vi "Needle Valve labVIEW Code.vi"() -> ()   [LabVIEW 2025]
uses:
  modesEnum.ctl
  <vilib>/Utility/file.llb/Read Delimited Spreadsheet (DBL).vi
  <vilib>/gmath/NI_Gmath.lvlib
  d3b0afdc-d7ac-4f1a-8ecc-0aeb21fe1e80.vi
  c8945bc9-af31-4a2e-9b52-27840c61c0f1.vi
  PIDController/PIDController.lvclass
  e7797c04-791b-4eea-89a1-5a3bec2431d3.vi
  bf5fd3a0-ddf8-478e-bb95-a39885d33854.vi
  0890acf7-df83-934e-a7ac-ae51bc85d557.vi
  d872897a-af24-4a4d-87bc-a1bb59a840a8.vi
  0285ecf2-4d18-4427-ace1-61b1951a0741.vi
  <vilib>/Instr/_visa.llb/VISA Configure Serial Port (Instr).vi
  <vilib>/Utility/file.llb/Write Delimited Spreadsheet (string).vi
  spikeController/spikeController.lvclass
panel:
  out "last error":dbl
  in  "Use D1":bool
  in  "Use D2":bool
  in  "Use Avg":bool
  in  "Save Graphs":bool
  in  "Set setPoint":dbl format="%.3f"
  in  "Set Spike Position":dbl format="%.3f"
  in  "setPoint":dbl(knob) scale=0.0..1000.0
  in  "A_max":dbl=6.5
  in  "A_min":dbl
  in  "k_i":dbl
  in  "k_d":dbl
  in  "k_p":dbl
  out "SafetyClose":bool
  out "PID":bool
  out "Manual":bool
  out "Idle":bool
  out "Ducer1":bool
  out "Ducer2":bool
  out "Avg Ducers":bool
  out "Read Pressure Ducer":dbl
  out "Raw Pressure Ducer 2":dbl
  in  "spikeController.lvclass":refnum<class "spikeController.lvclass">
  out "underAmin":bool
  out "overAmax":bool
  out "PID Output":dbl[](graph)
  out "PID Translated Output":dbl
  out "PID Output":dbl
  in  "loop stop 2":bool
  in  "loop stop 1":bool
  in  "PIDController.lvclass":refnum<class "PIDController.lvclass">
  out "VISA resource name out":refnum<visa-resource-name>
  in  "?":u32(colorbox)
  out "Reading Pressure Sensor":dbl[](graph)
  in  "?":dbl
  out "Motor Signal":string
  in  "stop program":bool
  in  "return spike":bool
  out "Spike Position \n(via Potentiometer)":dbl[](graph)
  out "Arduino Error":errorcluster
  in  "VISA resource Port":refnum<visa-resource-name>
  out "distance to go":dbl caption="Distance to Go (in)\n(For Reference Only)" format="%.3f"
  out "spike position":dbl format="%.3f"
  in  "Set Spike Position (in)":dbl(slide) scale=0.0..6.8
  out "?":dbl(slide) scale=0.0..1000.0
  out "Stagnation Flow Temp (K)\n(For Refrence only)":dbl
  out "Raw Pressure Ducer":dbl
  in  "Sensor Offsets":dbl[](array[numeric])=[10.0, 10.0, 0.0, 22.0]
  in  "Sensor K-values":dbl[](array[numeric])=[10.0, 10.0, 0.0, 22.0]
  in  "Exit PID Mode":bool
  in  "manual exit button":bool
  in  "Motor Control Loop Rate (ms)":dbl
  out "Set Motor RPM":dbl(knob) scale=0.0..200.0
  in  "PID Mode":bool
  in  "Manual Positioning Mode":bool
  in  "Stop Sensors":bool
  in  "Sensor Loop Rate (ms)":dbl
  out "Time Since Start (s)\n(For Reference Only)":dbl format="%.2f"
  in  "Start Sensors":bool
  in  "Load Inputs":bool
  in  "Save Inputs":bool
  out "Potentiometer distance":dbl
  out "Port":i32
  out "ConnectionType":i32
  out "DeviceType":i32
  out "Labjack error":errorcluster
  # "34HS59-6004S Motor Torque Curve (For Reference)"
  # "Labjack/Arduino Resources"
  # "Inputs and LabJack Sensor Monitors"
  # "PID Inputs"
  # "Motor RPM >200 RPM"
  # "Potentiometer"
  # "Inefficent Torque for High Mass Flow/Thrust Tests"
  # "Ducer"
  # "Thermocouple"
  # "Motor RPM < 200 RPM"
  # "(Labjack Auto-Populates)"
  # "(dial indicator for range reference)"
  # "COM Port for Arduino"
  # "Stop sensors automatically saves sensor data"
  # "Needliest"
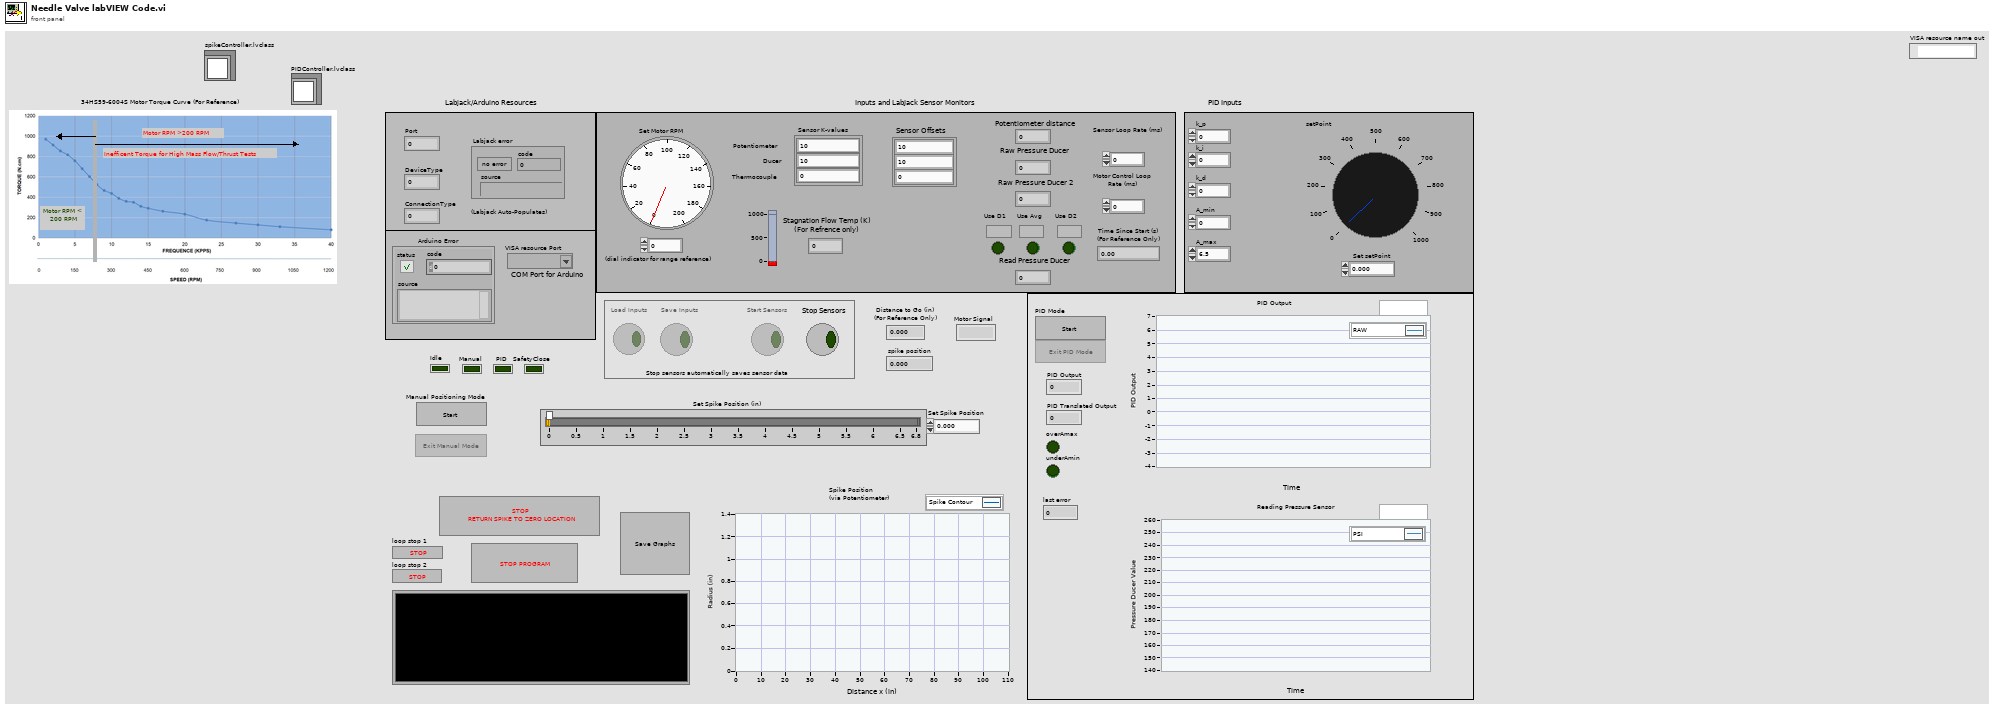
[diagram p1: front panel]
types:
  T1 = typedef "modesEnum.ctl" = enum16{"SafetyOpen", "SafetyClose", "SaveFile", "PIDControl", "ManualControl", "Idle"}
  T2 = enum8{"Enabled", "Disabled", "Disabled and Grayed Out"}
  T3 = enum16{"Potentiometer", "Ducer", "Thermocouple", "Ducer2"}
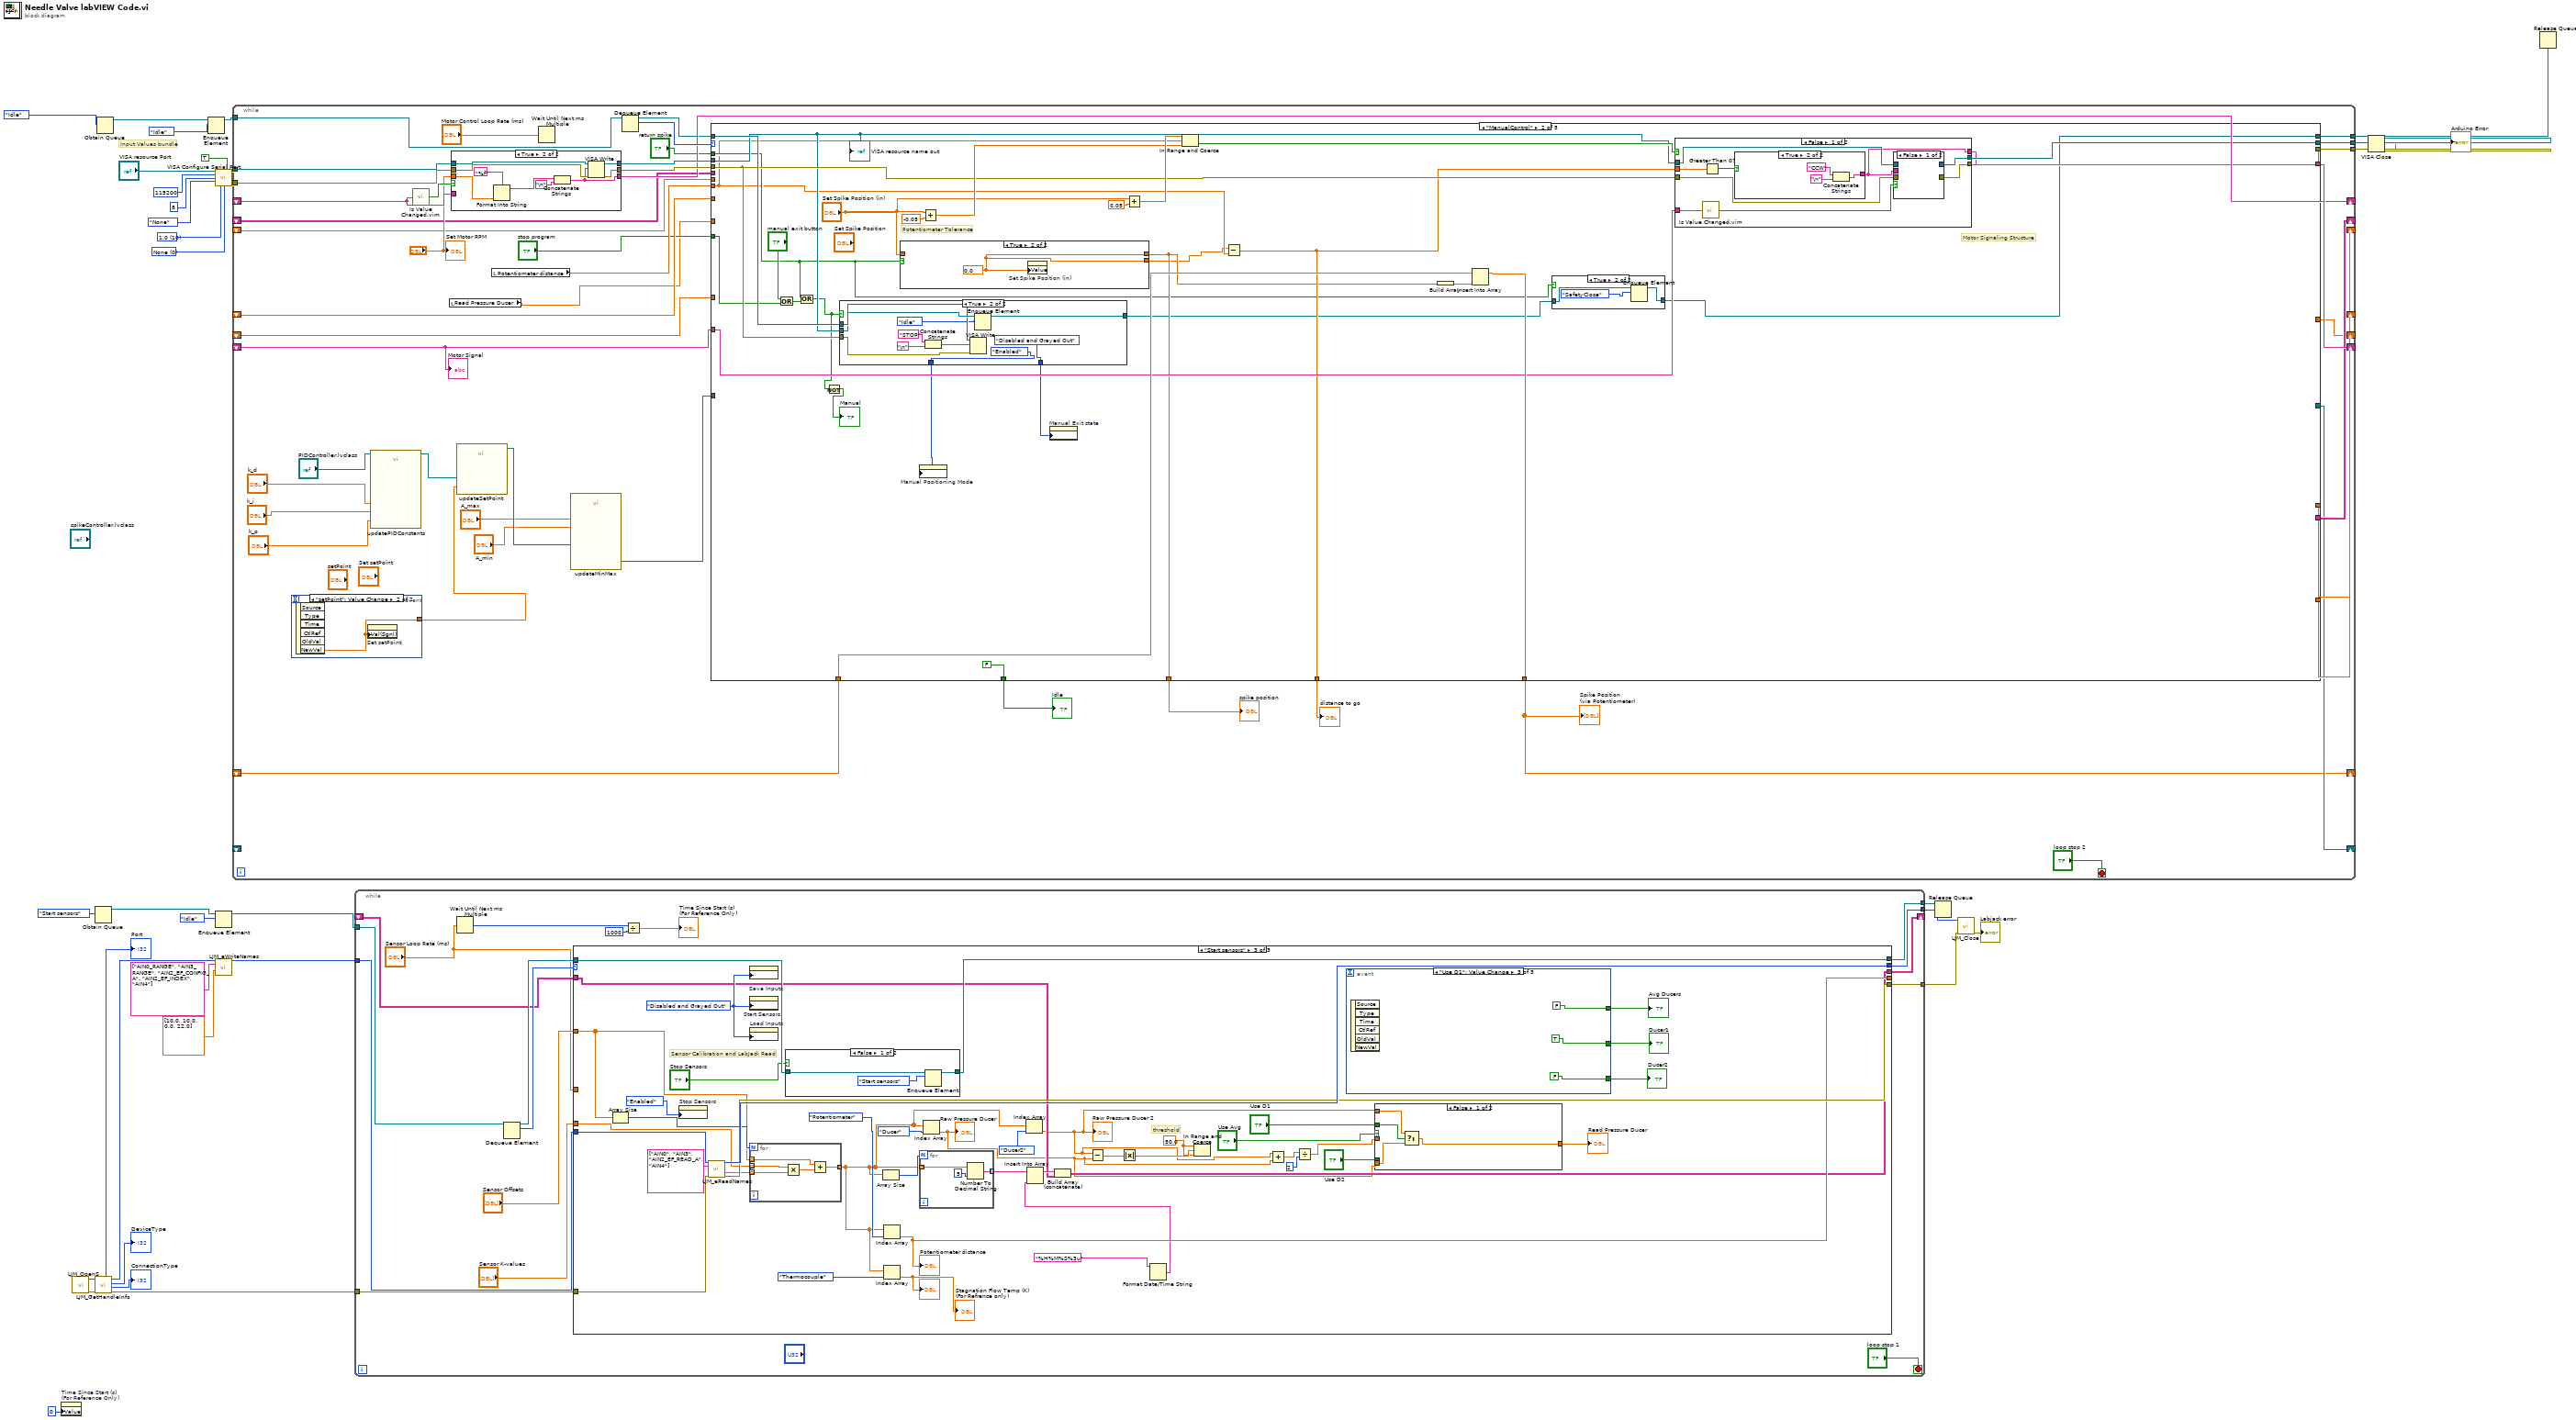
[diagram p0: block diagram]
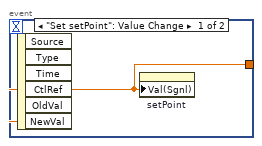
[diagram p2: hidden frame]
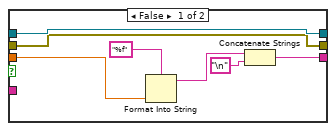
[diagram p3: hidden frame]
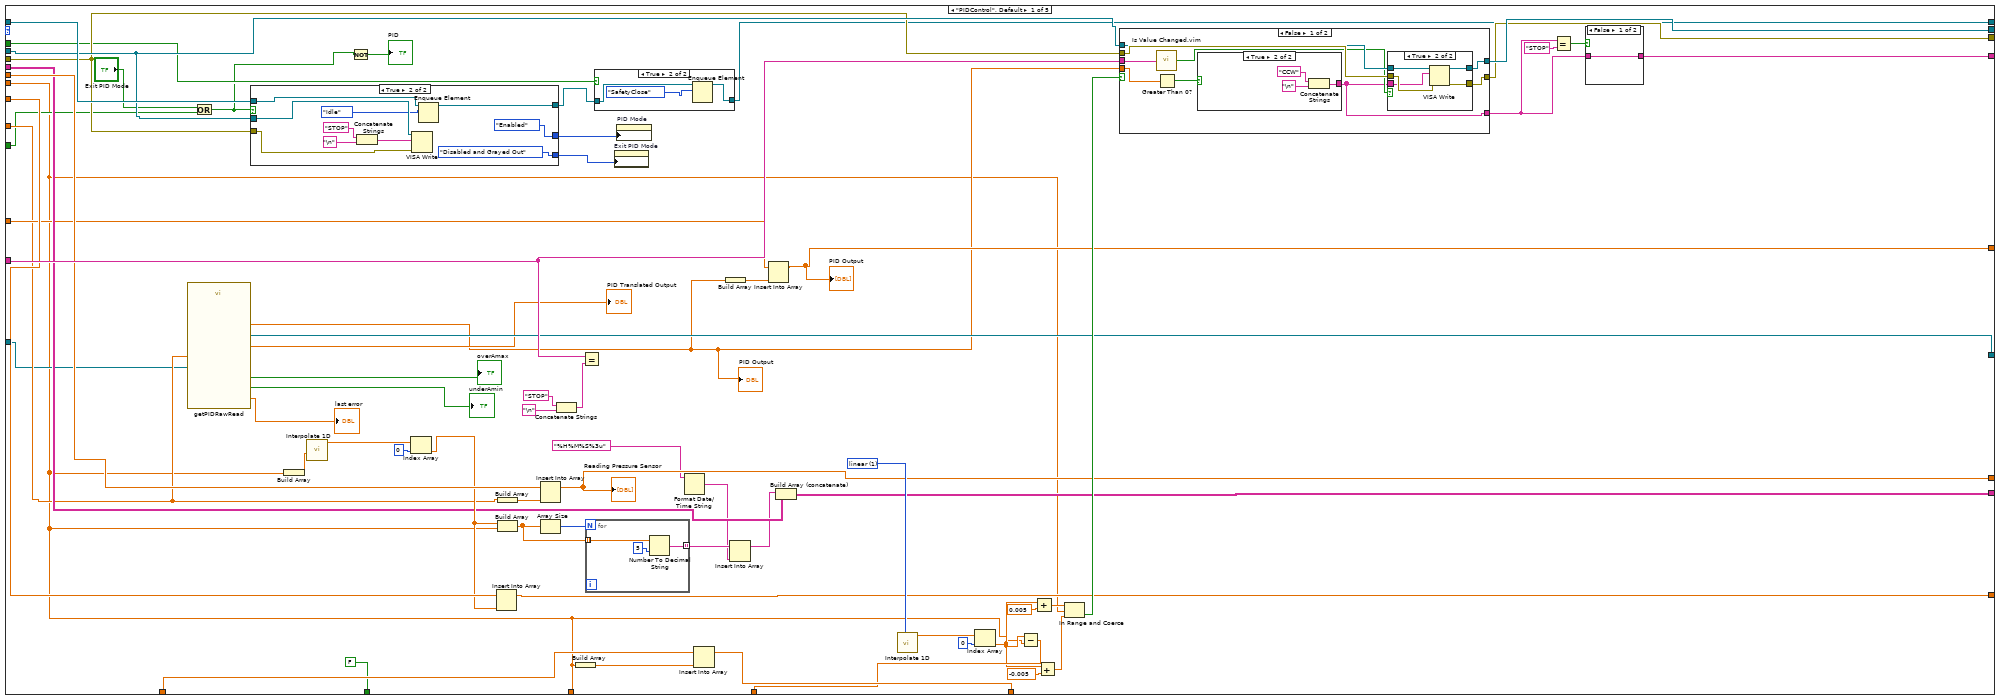
[diagram p4: hidden frame]
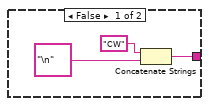
[diagram p8: hidden frame]
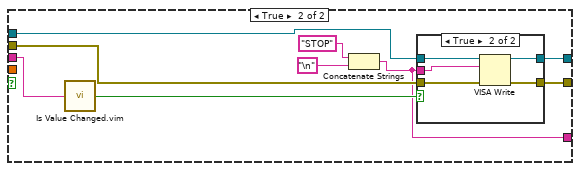
[diagram p9: hidden frame]
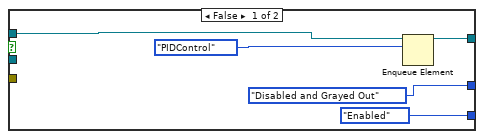
[diagram p11: hidden frame]
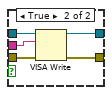
[diagram p14: hidden frame]
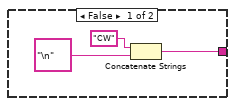
[diagram p15: hidden frame]
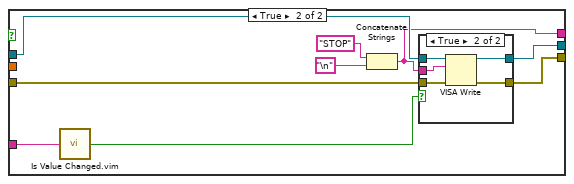
[diagram p16: hidden frame]
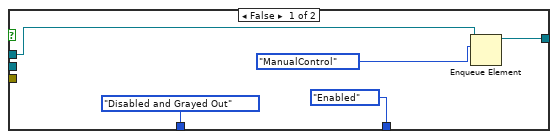
[diagram p18: hidden frame]
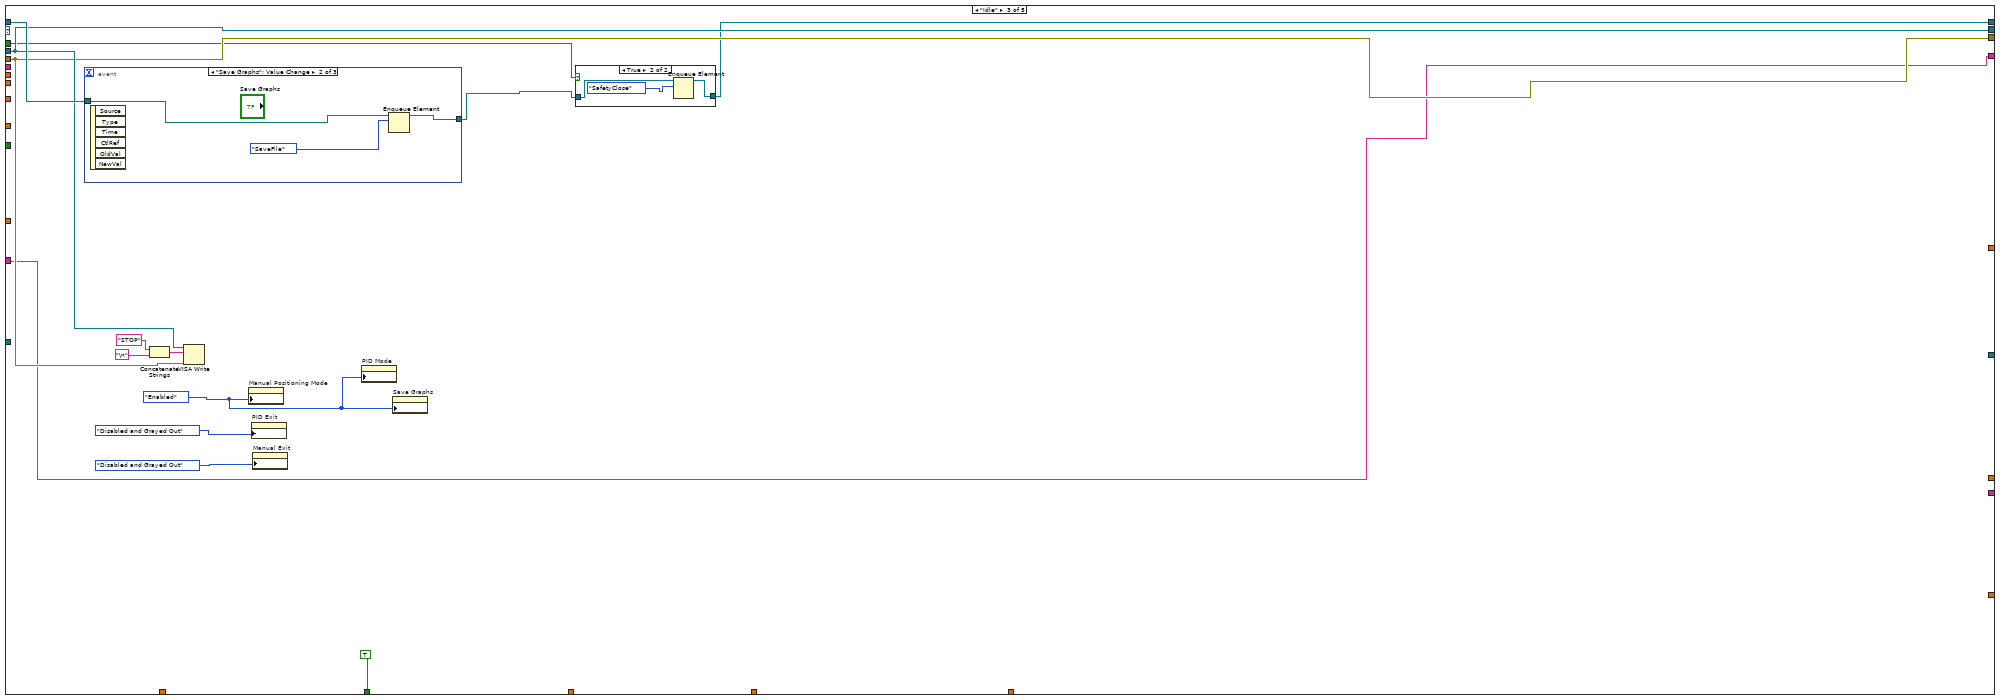
[diagram p19: hidden frame]
diagram:
  w6 = u16 0 items=["None", "XON/XOFF", "RTS/CTS", "XON/XOFF & RTS/CTS", "DTR/DSR", "XON/XOFF & DTR/DSR"] ("flow control (0:none)")
  w7 = u16 10 items=["1.0"=10, "1.5"=15, "2.0"=20] ("stop bits (10: 1 bit)")
  # "Input Values bundle"
  n1 = property on="Time Since Start (s)\n(For Reference Only)" class="DigNum (strict)"("Value"=u32 0 ("Time Since Start (s)\n(For Reference Only) 2")) -> ()  [unwired: 2 in, 2 out]
  n2 = call "LJM_OpenS.vi"() -> ("error out"=w31:errorcluster, "Handle"=w35:i32)  [unwired: 10 in]
  n3 = Obtain Queue(element data type=enum16{"Start sensors", "load Values", "Idle"}."Start sensors" ("Enum")) -> (queue out=w25:refnum<queue>)  [unwired: 4 in, 2 out]
  n4 = call "LJM_GetHandleInfo.vi"("error in"=w31, "Handle In"=w35) -> ("error out"=w30:errorcluster, "ConnectionType"=→"ConnectionType":i32, "DeviceType"=→"DeviceType":i32, "Handle Out"=w18:i32, "Port"=→"Port":i32)  [unwired: 2 in, 3 out]
  n5 = Obtain Queue(element data type=modesEnum."Idle" ("modesEnum")) -> (queue out=w27:refnum<queue>)  [unwired: 4 in, 2 out]
  n6 = Enqueue Element(queue=w27, element=modesEnum."Idle" ("modesEnum")) -> (queue out=w26:refnum<queue>)  [unwired: 2 in, 2 out]
  n7 = call-poly "VISA Configure Serial Port"("VISA resource name"="VISA resource Port", "Enable Termination\nChar (T)"=TRUE ("Enable Termination\nChar (T)"), "baud rate (9600)"=u32 115200, "data bits (8)"=u16 8, "parity (0:none)"=enum16{"None", "Odd", "Even", "Mark", "Space"}."None", "stop bits (10: 1 bit)"=w7, "flow control (0:none)"=w6) -> ("VISA resource name out"=w4:refnum<visa-resource-name>, "error out"=w5:errorcluster)  [unwired: 7 in]
  n8 = Enqueue Element(queue=w25, element=enum16{"Start sensors", "load Values", "Idle"}."Idle" ("Enum")) -> (queue out=w24:refnum<queue>)  [unwired: 2 in, 2 out]
  n9 = call "LJM_eWriteNames.vi"("Handle In"=w18, "aNames"=string[] ["AIN0_RANGE", "AIN3_RANGE", "AIN2_EF_CONFIG_A", "AIN2_EF_INDEX", "AIN4"], "aValuesIn"=dbl[] [10.0, 10.0, 0.0, 22.0]) -> ("Handle Out"=w17:i32)  [unwired: 10 in, 2 out]
  n10 = while {
    tunnel: w26 -> [w82]
    tunnel: [w80] -> w21
    tunnel: [w77] -> w12
    tunnel: [w76] -> w11
    shift-right: [w75] -> _
    shift-left: _ -> [w74]
    tunnel: w5 -> [w73]
    tunnel: w4 -> [w72]
    shift-right: [w68] -> _
    shift-left: _ -> [w67]
    shift-right: [w59] -> _
    shift-left: _ -> [_]
    shift-right: [w64] -> _
    shift-left: _ -> [w63]
    shift-right: [w62] -> _
    shift-left: _ -> [w57]
    shift-right: [w61] -> _
    shift-left: _ -> [w60]
    shift-right: [w55] -> _
    shift-left: _ -> [w56]
    shift-right: [w52] -> _
    shift-left: _ -> [w53]
    stop <- "loop stop 2" stop-if-true
    n11 = event shown="[1] \"setPoint\": Value Change" {
      selector: _ -> [_ _]
      dyn-events: _ -> [_ _]
      timeout: _ -> [_ _]
      tunnel: [w83 w84] -> w37
      event "Set setPoint": Value Change {
        n12 = event-data() -> ("NewVal"=w83:dbl)  [unwired: 1 in, 5 out]
        n13 = property on="setPoint" class="Knob (strict)"("Val(Sgnl)"=w83) -> ()  [unwired: 2 in, 2 out]
      }
      event "setPoint": Value Change {
        n14 = event-data() -> ("NewVal"=w84:dbl)  [unwired: 1 in, 5 out]
        n15 = property on="Set setPoint" class="DigNum (strict)"("Val(Sgnl)"=w84) -> ()  [unwired: 2 in, 2 out]
      }
    }
    n16 = call "updatePIDConstants.vi"("new k_d"="k_d", "new k_p"="k_p", "new k_i"="k_i", "PIDController in"="PIDController.lvclass") -> ("PIDController out"=w47:refnum<class "PIDController.lvclass">)  [unwired: 6 in, 1 out]
    n17 = call "Is Value Changed.vim"("value"=w67) -> ("changed or first call?"=w69:bool)
    n18 = local read "Read Pressure Ducer"() -> (w38:dbl)
    n19 = case shown="True" w69 {
      tunnel: w73 -> [w90 w100]
      tunnel: [w86 w92] -> w68
      tunnel: w72 -> [w91 w99]
      tunnel: [w90 w98] -> w71
      tunnel: [w91 w95] -> w70
      tunnel: "?" -> [w89 w97]
      tunnel: w67 -> [_ _]
      frame False {
        n20 = Format Into String(format string="%f", w89) -> (resulting string=w87:string)  [unwired: 2 in, 1 out]
        n21 = Concatenate Strings(w87, "\n" ("string")) -> (w86:string)
      }
      frame True {
        n22 = Format Into String(format string="%f", w97) -> (resulting string=w94:string)  [unwired: 2 in, 1 out]
        n23 = Concatenate Strings(w94, "\n" ("string")) -> (w92:string)
        n24 = VISA Write(VISA resource name=w99, write buffer=w92, error in (no error)=w100) -> (VISA resource name out=w95:refnum<visa-resource-name>, error out=w98:errorcluster)  [unwired: 1 out]
      }
    }
    n25 = call "updateSetPoint.vi"("new setpoint"=w37, "PIDController in"=w47) -> ("PIDController out"=w48:refnum<class "PIDController.lvclass">)  [unwired: 8 in, 1 out]
    n26 = local read "Potentiometer distance"() -> (w78:dbl)
    n27 = Wait Until Next ms Multiple(millisecond multiple="Motor Control Loop Rate (ms)") -> ()  [unwired: 1 out]
    n28 = call "updateMinMax.vi"("a_max"="A_max", "a_min"="A_min", "PIDController in"=w48) -> ("PIDController out"=w45:refnum<class "PIDController.lvclass">)  [unwired: 7 in, 1 out]
    n29 = Dequeue Element(queue=w82) -> (queue out=w49:refnum<queue>, element=w81:T1)  [unwired: 2 in, 2 out]
    n30 = case shown="\"ManualControl\"" w81 {
      tunnel: [w111 w231 w314 w347 _] -> w80
      tunnel: w49 -> [w165 w254 w323 w346 _]
      tunnel: w78 -> [w107 w230 _ w341 _]
      tunnel: w70 -> [w154 w243 w317 w351 _]
      tunnel: [w157 w248 w317 w349 _] -> w77
      tunnel: w71 -> [w153 w245 w316 w352 _]
      tunnel: [w156 w247 w316 w348 _] -> w76
      tunnel: [w150 w246 w315 w350 _] -> w75
      tunnel: w74 -> [w148 w236 w315 w340 _]
      tunnel: "return spike" -> [w110 w233 w312 w339 _]
      tunnel: [w140 _ _ _ _] -> w64
      tunnel: w63 -> [w141 _ _ _ _]
      tunnel: [w138 _ _ _ _] -> w62
      tunnel: w57 -> [w137 _ _ _ w399]
      tunnel: [w134 _ _ _ _] -> w61
      tunnel: w60 -> [w133 _ _ _ _]
      tunnel: w38 -> [w121 _ _ _ _]
      tunnel: w45 -> [w109 _ _ _ _]
      tunnel: [w127 _ _ _ _] -> w59
      tunnel: w56 -> [w125 _ _ _ w398]
      tunnel: [w124 _ _ _ _] -> w55
      tunnel: "stop program" -> [w117 w241 _ _ _]
      tunnel: w53 -> [w115 w238 _ w345 w419]
      tunnel: [w114 w237 _ w344 _] -> w52
      tunnel: [w113 w235 _ w343 _] -> w51
      tunnel: [w107 w234 _ w342 _] -> w50
      tunnel: [FALSE FALSE TRUE FALSE FALSE] -> w39
      frame "PIDControl", Default {
        w158 = 1 items=["nearest", "linear", "spline", "cubic Hermite", "Lagrange"] ("method")
        n31 = call "getPIDRawRead.vi"("sensorValue"=w121, "PIDController in"=w109) -> ("overAmin"=→"underAmin":bool, "translatedPIDOutput"=→"PID Translated Output":dbl, "PIDRawRead"=w123:dbl, "PIDController out"=w127:refnum<class "PIDController.lvclass">, "underAmax"=→"overAmax":bool, "lastErrorRead"=→"last error":dbl)  [unwired: 4 in]
        "PID Output" <- w123
        n32 = Or(x="Exit PID Mode", y=w117) -> (x .or. y?=w106:bool)
        n33 = case shown="True" w106 {
          tunnel: w165 -> [w213 w223]
          tunnel: [w212 w222] -> w112
          tunnel: w154 -> [_ w218]
          tunnel: w153 -> [_ w217]
          tunnel: [T2."Disabled and Grayed Out" ("Disabled") T2."Enabled" ("Disabled")] -> w103
          tunnel: [T2."Enabled" ("Disabled") T2."Disabled and Grayed Out" ("Disabled")] -> w102
          frame False {
            n34 = Enqueue Element(queue=w213, element=modesEnum."PIDControl" ("modesEnum")) -> (queue out=w212:refnum<queue>)  [unwired: 2 in, 2 out]
          }
          frame True {
            n35 = Concatenate Strings("STOP" ("write buffer"), "\n" ("write buffer")) -> (w221:string)
            n36 = VISA Write(VISA resource name=w218, write buffer=w221, error in (no error)=w217) -> ()  [unwired: 3 out]
            n37 = Enqueue Element(queue=w223, element=modesEnum."Idle" ("modesEnum")) -> (queue out=w222:refnum<queue>)  [unwired: 2 in, 2 out]
          }
        }
        n38 = Build Array(w107) -> (w147:dbl[])
        n39 = call <vilib>:"Interpolate 1D.vi"("xi"=w147) -> ("yi"=w146:dbl[])  [unwired: 8 in, 2 out]
        n40 = Not(x=w106) -> (.not. x?=→"PID":bool)
        n41 = Index Array(array=w146, index=0) -> (element=w136:dbl)
        n42 = Insert Into Array(array=w141, new element=w136) -> (w140:dbl[])  [unwired: 1 in]
        n43 = Build Array(w121) -> (w139:dbl[])
        n44 = Build Array(w136, w107) -> (w132:dbl[])
        n45 = Insert Into Array(array=w137, new element=w139) -> (w138:dbl[])  [unwired: 1 in]
        "Reading Pressure Sensor" <- w138
        n46 = Array Size(array=w132) -> (size(s)=w131:i32)
        n47 = Concatenate Strings("STOP" ("string"), "\n" ("string")) -> (w142:string)
        n48 = Build Array(w107) -> (w116:dbl[])
        n49 = Equal?(x=w148, y=w142) -> ()  [unwired: 1 out]
        n50 = for {
          N: w131 -> [_]
          tunnel: w132 -> [w172] mode=indexing
          tunnel: [w170] -> w135 mode=indexing
          n51 = Number To Decimal String(number=w172, width (-)=i16 5) -> (decimal integer string=w170:string)
        }
        n52 = case shown="True" w110 {
          tunnel: w112 -> [w166 w169]
          tunnel: [w166 w168] -> w111
          frame False {
          }
          frame True {
            n53 = Enqueue Element(queue=w169, element=modesEnum."SafetyClose" ("modesEnum")) -> (queue out=w168:refnum<queue>)  [unwired: 2 in, 2 out]
          }
        }
        n54 = property on="Exit PID Mode" class="Bool"("DisabledEnum"=w102) -> ()  [unwired: 2 in, 2 out]
        n55 = property on="PID Mode" class="Bool"("DisabledEnum"=w103) -> ()  [unwired: 2 in, 2 out]
        n56 = Format Date/Time String(time format string (%c)="%H%M%S%3u") -> (date/time string=w128:string)  [unwired: 2 in]
        n57 = Insert Into Array(array=w115, new element=w116) -> (w114:dbl[])  [unwired: 1 in]
        n58 = Build Array(w123) -> (w122:dbl[])
        n59 = Insert Into Array(array=w135, new element=w128) -> (w130:string[])  [unwired: 1 in]
        n60 = Insert Into Array(array=w125, new element=w122) -> (w124:dbl[])  [unwired: 1 in]
        "PID Output" <- w124
        n61 = Build Array (concatenate)(w130, w133) -> (w134:string[][])
        n62 = call <vilib>:"Interpolate 1D.vi"("method"=w158) -> ("yi"=w159:dbl[])  [unwired: 8 in, 2 out]
        n63 = Index Array(array=w159, index=0) -> (element=w108:dbl)
        n64 = Subtract(x=w108, y=w107) -> (x-y=w113:dbl)
        n65 = Add(x=w108, y=0.005) -> (x+y=w164:dbl)
        n66 = Add(x=w108, y=-0.005) -> (x+y=w162:dbl)
        n67 = In Range and Coerce(upper limit=w164, x=w107, lower limit=w162) -> (In Range?=w155:bool)  [unwired: 1 out]
        n68 = case shown="False" w155 {
          tunnel: w123 -> [w182 _]
          tunnel: w154 -> [w180 w203]
          tunnel: [w178 w200] -> w157
          tunnel: w153 -> [w181 w199]
          tunnel: [w179 w198] -> w156
          tunnel: [w175 w195] -> w151
          tunnel: w148 -> [w177 w202]
          frame False {
            n69 = call "Is Value Changed.vim"("value"=w177) -> ("changed or first call?"=w176:bool)
            n70 = Greater Than 0?(x=w182) -> (x > 0?=w183:bool)
            n71 = case shown="True" w183 {
              tunnel: [w189 w192] -> w175
              frame False {
                n72 = Concatenate Strings("CW" ("write buffer"), "\n" ("write buffer")) -> (w189:string)
              }
              frame True {
                n73 = Concatenate Strings("CCW" ("write buffer"), "\n" ("write buffer")) -> (w192:string)
              }
            }
            n74 = case shown="True" w176 {
              tunnel: w181 -> [_ w188]
              tunnel: w180 -> [_ w187]
              tunnel: [_ w186] -> w179
              tunnel: [_ w185] -> w178
              tunnel: w175 -> [_ w184]
              frame False {
              }
              frame True {
                n75 = VISA Write(VISA resource name=w187, write buffer=w184, error in (no error)=w188) -> (VISA resource name out=w185:refnum<visa-resource-name>, error out=w186:errorcluster)  [unwired: 1 out]
              }
            }
          }
          frame True {
            n76 = call "Is Value Changed.vim"("value"=w202) -> ("changed or first call?"=w201:bool)
            n77 = Concatenate Strings("STOP" ("write buffer"), "\n" ("write buffer")) -> (w195:string)
            n78 = case shown="True" w201 {
              tunnel: w195 -> [_ w208]
              tunnel: w203 -> [_ w207]
              tunnel: [_ w206] -> w200
              tunnel: w199 -> [_ w205]
              tunnel: [_ w204] -> w198
              frame False {
              }
              frame True {
                n79 = VISA Write(VISA resource name=w207, write buffer=w208, error in (no error)=w205) -> (VISA resource name out=w206:refnum<visa-resource-name>, error out=w204:errorcluster)  [unwired: 1 out]
              }
            }
          }
        }
        n80 = Equal?(x=w151, y="STOP" ("write buffer")) -> (x = y?=w149:bool)
        n81 = case shown="False" w149 {
          tunnel: [w173 w174] -> w150
          tunnel: w151 -> [w173 w174]
          frame False {
          }
          frame True {
          }
        }
      }
      frame "ManualControl" {
        # "Motor Signaling Structure"
        # "Potentiometer Tolerance"
        n82 = Or(x="manual exit button", y=w241) -> (x .or. y?=w240:bool)
        n83 = Or(x=w233, y=w240) -> (x .or. y?=w228:bool)
        n84 = Not(x=w228) -> (.not. x?=→"Manual":bool)
        n85 = case shown="True" w228 {
          tunnel: w254 -> [w299 w309]
          tunnel: [w298 w308] -> w232
          tunnel: w243 -> [_ w304]
          tunnel: w245 -> [_ w303]
          tunnel: [T2."Enabled" ("Disabled") T2."Disabled and Grayed Out" ("Disabled")] -> w225
          tunnel: [T2."Disabled and Grayed Out" ("Disabled") T2."Enabled" ("Disabled")] -> w224
          frame False {
            n86 = Enqueue Element(queue=w299, element=modesEnum."ManualControl" ("modesEnum")) -> (queue out=w298:refnum<queue>)  [unwired: 2 in, 2 out]
          }
          frame True {
            n87 = Concatenate Strings("STOP" ("write buffer"), "\n" ("write buffer")) -> (w307:string)
            n88 = VISA Write(VISA resource name=w304, write buffer=w307, error in (no error)=w303) -> ()  [unwired: 3 out]
            n89 = Enqueue Element(queue=w309, element=modesEnum."Idle" ("modesEnum")) -> (queue out=w308:refnum<queue>)  [unwired: 2 in, 2 out]
          }
        }
        n90 = case shown="True" w233 {
          tunnel: [w259 w260] -> w229
          tunnel: "Set Spike Position (in)" -> [w259 _]
          tunnel: [w259 w260] -> w234
          frame False {
          }
          frame True {
            w260 = 0.0
            n91 = property on="Set Spike Position (in)" class="Slide (strict)"("Value"=w260) -> ()  [unwired: 2 in, 2 out]
          }
        }
        n92 = property on="Manual Positioning Mode" class="Bool"("DisabledEnum"=w224) -> ()  [unwired: 2 in, 2 out]
        n93 = Add(x="Set Spike Position (in)", y=-0.05) -> (x+y=w250:dbl)
        n94 = property on="Manual Exit state" class="Bool"("DisabledEnum"=w225) -> ()  [unwired: 2 in, 2 out]
        n95 = Add(x="Set Spike Position (in)", y=0.05) -> (x+y=w252:dbl)
        n96 = In Range and Coerce(upper limit=w252, x=w230, lower limit=w250) -> (In Range?=w253:bool)  [unwired: 1 out]
        n97 = Subtract(x=w229, y=w230) -> (x-y=w235:dbl)
        n98 = Build Array(w234) -> (w239:dbl[])
        n99 = Insert Into Array(array=w238, new element=w239) -> (w237:dbl[])  [unwired: 1 in]
        n100 = case shown="True" w233 {
          tunnel: w232 -> [w255 w258]
          tunnel: [w255 w257] -> w231
          frame False {
          }
          frame True {
            n101 = Enqueue Element(queue=w258, element=modesEnum."SafetyClose" ("modesEnum")) -> (queue out=w257:refnum<queue>)  [unwired: 2 in, 2 out]
          }
        }
        n102 = case shown="False" w253 {
          tunnel: w235 -> [w268 _]
          tunnel: w243 -> [w266 w289]
          tunnel: [w264 w286] -> w248
          tunnel: w245 -> [w267 w285]
          tunnel: [w265 w284] -> w247
          tunnel: [w261 w281] -> w246
          tunnel: w236 -> [w263 w288]
          frame False {
            n103 = call "Is Value Changed.vim"("value"=w263) -> ("changed or first call?"=w262:bool)
            n104 = Greater Than 0?(x=w268) -> (x > 0?=w269:bool)
            n105 = case shown="True" w269 {
              tunnel: [w275 w278] -> w261
              frame False {
                n106 = Concatenate Strings("CW" ("write buffer"), "\n" ("write buffer")) -> (w275:string)
              }
              frame True {
                n107 = Concatenate Strings("CCW" ("write buffer"), "\n" ("write buffer")) -> (w278:string)
              }
            }
            n108 = case shown="False" w262 {
              tunnel: w267 -> [_ w274]
              tunnel: w266 -> [_ w273]
              tunnel: [_ w272] -> w265
              tunnel: [_ w271] -> w264
              tunnel: w261 -> [_ w270]
              frame False {
              }
              frame True {
                n109 = VISA Write(VISA resource name=w273, write buffer=w270, error in (no error)=w274) -> (VISA resource name out=w271:refnum<visa-resource-name>, error out=w272:errorcluster)  [unwired: 1 out]
              }
            }
          }
          frame True {
            n110 = call "Is Value Changed.vim"("value"=w288) -> ("changed or first call?"=w287:bool)
            n111 = Concatenate Strings("STOP" ("write buffer"), "\n" ("write buffer")) -> (w281:string)
            n112 = case shown="True" w287 {
              tunnel: w281 -> [_ w294]
              tunnel: w289 -> [_ w293]
              tunnel: [_ w292] -> w286
              tunnel: w285 -> [_ w291]
              tunnel: [_ w290] -> w284
              frame False {
              }
              frame True {
                n113 = VISA Write(VISA resource name=w293, write buffer=w294, error in (no error)=w291) -> (VISA resource name out=w292:refnum<visa-resource-name>, error out=w290:errorcluster)  [unwired: 1 out]
              }
            }
          }
        }
        "VISA resource name out" <- w243
      }
      frame "Idle" {
        w310 = T2."Enabled" ("Disabled")
        n114 = event shown="[1] \"Save Graphs\": Value Change" {
          selector: _ -> [_ _ _]
          dyn-events: _ -> [_ _ _]
          timeout: _ -> [_ _ _]
          tunnel: w323 -> [w330 w333 w336]
          tunnel: [w329 w332 w335] -> w313
          event "Manual Positioning Mode": Value Change {
            n115 = event-data() -> ()  [unwired: 1 in, 6 out]
            n116 = Enqueue Element(queue=w330, element=modesEnum."ManualControl" ("modesEnum")) -> (queue out=w329:refnum<queue>)  [unwired: 2 in, 2 out]
          }
          event "Save Graphs": Value Change {
            n117 = event-data() -> ()  [unwired: 1 in, 6 out]
            n118 = Enqueue Element(queue=w333, element=modesEnum."SaveFile" ("modesEnum")) -> (queue out=w332:refnum<queue>)  [unwired: 2 in, 2 out]
          }
          event "PID Mode": Value Change {
            n119 = event-data() -> ()  [unwired: 1 in, 6 out]
            n120 = Enqueue Element(queue=w336, element=modesEnum."PIDControl" ("modesEnum")) -> (queue out=w335:refnum<queue>)  [unwired: 2 in, 2 out]
          }
        }
        n121 = Concatenate Strings("STOP" ("write buffer"), "\n" ("write buffer")) -> (w320:string)
        n122 = VISA Write(VISA resource name=w317, write buffer=w320, error in (no error)=w316) -> ()  [unwired: 3 out]
        n123 = property on="Manual Positioning Mode" class="Bool"("DisabledEnum"=w310) -> ()  [unwired: 2 in, 2 out]
        n124 = property on="PID Exit" class="Bool"("DisabledEnum"=T2."Disabled and Grayed Out" ("Disabled")) -> ()  [unwired: 2 in, 2 out]
        n125 = property on="Manual Exit" class="Bool"("DisabledEnum"=T2."Disabled and Grayed Out" ("Disabled")) -> ()  [unwired: 2 in, 2 out]
        n126 = property on="PID Mode" class="Bool"("DisabledEnum"=w310) -> ()  [unwired: 2 in, 2 out]
        n127 = property on="Save Graphs" class="Bool"("DisabledEnum"=w310) -> ()  [unwired: 2 in, 2 out]
        n128 = case shown="True" w312 {
          tunnel: w313 -> [w324 w325]
          tunnel: [w324 w327] -> w314
          frame False {
          }
          frame True {
            n129 = Enqueue Element(queue=w325, element=modesEnum."SafetyClose" ("modesEnum")) -> (queue out=w327:refnum<queue>)  [unwired: 2 in, 2 out]
          }
        }
      }
      frame "SafetyClose" {
        (unwired) T2."Disabled and Grayed Out" ("Disabled")
        (unwired) T2."Disabled and Grayed Out" ("Disabled")
        (unwired) T2."Disabled and Grayed Out" ("Disabled")
        w337 = T2."Disabled and Grayed Out" ("Disabled")
        w342 = 0.0
        # "Motor Signaling Structure"
        # "Potentiometer Tolerance"
        n130 = property on="Manual Positioning Mode" class="Bool"("DisabledEnum"=w337) -> ()  [unwired: 2 in, 2 out]
        n131 = property on="manual exit button" class="Bool"("DisabledEnum"=w337) -> ()  [unwired: 2 in, 2 out]
        n132 = property on="Exit PID Mode" class="Bool"("DisabledEnum"=w337) -> ()  [unwired: 2 in, 2 out]
        n133 = property on="PID Mode" class="Bool"("DisabledEnum"=w337) -> ()  [unwired: 2 in, 2 out]
        n134 = Add(x=w341, y=-0.005) -> (x+y=w355:dbl)
        n135 = Add(x=w341, y=0.005) -> (x+y=w357:dbl)
        n136 = In Range and Coerce(upper limit=w357, x=w341, lower limit=w355) -> (In Range?=w358:bool)  [unwired: 1 out]
        n137 = Subtract(x=w341, y=w342) -> (x-y=w343:dbl)
        n138 = Build Array(w342) -> (w353:dbl[])
        n139 = Insert Into Array(array=w345, new element=w353) -> (w344:dbl[])  [unwired: 1 in]
        n140 = case shown="False" w358 {
          tunnel: w343 -> [w366 _]
          tunnel: w351 -> [w364 w390]
          tunnel: [w362 w387] -> w349
          tunnel: w352 -> [w365 w386]
          tunnel: [w363 w385] -> w348
          tunnel: [w359 w382] -> w350
          tunnel: w340 -> [w361 w389]
          tunnel: w346 -> [_ w381]
          tunnel: [_ w380] -> w347
          frame False {
            n141 = call "Is Value Changed.vim"("value"=w361) -> ("changed or first call?"=w360:bool)
            n142 = Greater Than 0?(x=w366) -> (x > 0?=w367:bool)
            n143 = case shown="True" w367 {
              tunnel: [w373 w376] -> w359
              frame False {
                n144 = Concatenate Strings("CW" ("write buffer"), "\n" ("write buffer")) -> (w373:string)
              }
              frame True {
                n145 = Concatenate Strings("CCW" ("write buffer"), "\n" ("write buffer")) -> (w376:string)
              }
            }
            n146 = case shown="True" w360 {
              tunnel: w365 -> [_ w372]
              tunnel: w364 -> [_ w371]
              tunnel: [_ w370] -> w363
              tunnel: [_ w369] -> w362
              tunnel: w359 -> [_ w368]
              frame False {
              }
              frame True {
                n147 = VISA Write(VISA resource name=w371, write buffer=w368, error in (no error)=w372) -> (VISA resource name out=w369:refnum<visa-resource-name>, error out=w370:errorcluster)  [unwired: 1 out]
              }
            }
          }
          frame True {
            n148 = call "Is Value Changed.vim"("value"=w389) -> ("changed or first call?"=w388:bool)
            n149 = Enqueue Element(queue=w381, element=modesEnum."Idle" ("modesEnum")) -> (queue out=w380:refnum<queue>)  [unwired: 2 in, 2 out]
            n150 = Concatenate Strings("STOP" ("write buffer"), "\n" ("write buffer")) -> (w382:string)
            n151 = case shown="True" w388 {
              tunnel: w382 -> [_ w395]
              tunnel: w390 -> [_ w394]
              tunnel: [_ w393] -> w387
              tunnel: w386 -> [_ w392]
              tunnel: [_ w391] -> w385
              frame False {
              }
              frame True {
                n152 = VISA Write(VISA resource name=w394, write buffer=w395, error in (no error)=w392) -> (VISA resource name out=w393:refnum<visa-resource-name>, error out=w391:errorcluster)  [unwired: 1 out]
              }
            }
          }
        }
        "SafetyClose" <- w339
      }
      frame "SaveFile" {
        w396 = "%s"
        w397 = string[][] []
        # "PID"
        # "ducer"
        # "Pad arrays to same size"
        # "blanks"
        # "Spike Position"
        n153 = Array Size(array=w399) -> (size(s)=w423:i32)
        n154 = Array Size(array=w398) -> (size(s)=w425:i32)
        n155 = Array Size(array=w419) -> (size(s)=w426:i32)
        n156 = Max & Min(x=w426, y=w423) -> (max(x,y)=w427:i32)  [unwired: 1 out]
        n157 = Max & Min(x=w427, y=w425) -> (max(x,y)=w424:i32)  [unwired: 1 out]
        n158 = Subtract(x=w424, y=w426) -> (x-y=w421:i32)
        n159 = Subtract(x=w424, y=w425) -> (x-y=w411:i32)
        n160 = Subtract(x=w423, y=w424) -> (x-y=w412:i32)
        n161 = Array To Spreadsheet String(array=w398, 3:w396) -> (spreadsheet string=w434:string)  [unwired: 1 in]
        n162 = Array To Spreadsheet String(array=w399, 3:w396) -> (spreadsheet string=w400:string)  [unwired: 1 in]
        n163 = Array To Spreadsheet String(array=w419, 3:w396) -> (spreadsheet string=w436:string)  [unwired: 1 in]
        n164 = Initialize Array("", w411) -> (w413:string[])
        n165 = Initialize Array("", w412) -> (w415:string[])
        n166 = Initialize Array("", w421) -> (w420:string[])
        n167 = Spreadsheet String To Array(format string=w396, spreadsheet string=w400, array type (2D Dbl)=w397) -> (array=w410:string[][])  [unwired: 1 in]
        n168 = Spreadsheet String To Array(format string=w396, spreadsheet string=w436, array type (2D Dbl)=w397) -> (array=w418:string[][])  [unwired: 1 in]
        n169 = Spreadsheet String To Array(format string=w396, spreadsheet string=w434, array type (2D Dbl)=w397) -> (array=w408:string[][])  [unwired: 1 in]
        n170 = Build Array (concatenate)(w408, w413) -> (w407:string[][])
        n171 = Build Array (concatenate)(w410, w415) -> (w409:string[][])
        n172 = Build Array (concatenate)(w418, w420) -> (w417:string[][])
        n173 = Get Date/Time In Seconds() -> (seconds since 1Jan1904=w402:timestamp)
        n174 = Seconds To Date/Time(time stamp (now)=w402) -> ()  [unwired: 1 in, 1 out]
        n175 = Format Date/Time String(time format string (%c)="%Y-%m-%d_%H-%M-%S", seconds (now)=w402) -> (date/time string=w405:string)  [unwired: 1 in]
        n176 = Array Size(array=w417) -> (size(s)=w430:i32[])
        n177 = Index Array(array=w430, index=0) -> (element=w428:i32)
        n178 = Initialize Array("", w428, 1) -> (w435:string[][])
        n179 = Concatenate Strings("needleValveData_", w405) -> (w403:string)
        n180 = Build Array (concatenate)(string[] ["", "Time", "Spike Position", " ", "", "Time", "Pressure Ducer", "", "", "Time", "PID Output"], w417, w435, w435, w409, w435, w435, w407) -> (w437:string[][])
        n181 = call "File Dialog"("prompt"="Please Select Folder for Graph Data to be Saved", "default name"=w403) -> ("selected path"=w440:path)  [unwired: 10 in, 3 out]
        n182 = call-poly <vilib>:"Write Delimited Spreadsheet.vi"("file path (dialog if empty)"=w440, "2D data"=w437, "delimiter (\\t)"=",") -> ()  [unwired: 11 in, 2 out]
      }
    }
    "Spike Position \n(via Potentiometer)" <- w52
    "distance to go" <- w51
    "spike position" <- w50
    "Idle" <- w39
    "Set Motor RPM" <- "?"
    "Motor Signal" <- w74
  }
  n183 = while {
    tunnel: w30 -> [w457]
    tunnel: [w456] -> w29
    tunnel: w17 -> [w455]
    tunnel: [w454] -> w28
    tunnel: w24 -> [w453]
    tunnel: [w450] -> w22
    shift-right: [w444] -> _
    shift-left: _ -> [w443]
    stop <- "loop stop 1" stop-if-true
    n184 = Wait Until Next ms Multiple(millisecond multiple="Sensor Loop Rate (ms)") -> (millisecond timer value=w449:u32)
    n185 = Dequeue Element(queue=w453) -> (queue out=w451:refnum<queue>, element=w452:enum16{"Start sensors", "load Values", "Idle"})  [unwired: 2 in, 2 out]
    n186 = case shown="\"Start sensors\"" w452 {
      tunnel: w457 -> [_ _ w528]
      tunnel: [_ _ w527] -> w456
      tunnel: w455 -> [_ _ w530]
      tunnel: [_ _ w529] -> w454
      tunnel: w451 -> [w460 w483 w535]
      tunnel: [w459 w482 w534] -> w450
      tunnel: [_ _ w522] -> _
      tunnel: "Sensor Offsets" -> [_ _ w524]
      tunnel: "Sensor K-values" -> [_ _ w523]
      tunnel: [_ _ w516] -> w444
      tunnel: w443 -> [_ _ w515]
      tunnel: "Sensor Loop Rate (ms)" -> [_ _ _]
      frame "load Values" {
        n187 = flat-sequence {
          frame #0 {
            n188 = Two Button Dialog(message="Sensor and RPM File Selection" ("Message")) -> (T button?=w461:bool)  [unwired: 2 in]
            n189 = case shown="False" w461 {
              frame False {
              }
              frame True {
                # "Loading Motor RPM"
                n190 = call-poly <vilib>:"Read Delimited Spreadsheet.vi"() -> ("all rows"=w464:dbl[][])  [unwired: 10 in, 5 out]
                n191 = Index Array(array=w464, index (row)=0) -> (element=w478:dbl[])  [unwired: 1 in]
                n192 = Index Array(array=w464, index (row)=2) -> (element=w474:dbl[])  [unwired: 1 in]
                n193 = Index Array(array=w464, index (row)=1) -> (element=w476:dbl[])  [unwired: 1 in]
                n194 = property on="Sensor K-values" class="Arr (strict)"("Value"=w478) -> ()  [unwired: 2 in, 2 out]
                n195 = property on="Sensor Offsets" class="Arr (strict)"("Value"=w476) -> ()  [unwired: 2 in, 2 out]
                n196 = Index Array(array=w464, index (row)=3) -> (element=w470:dbl[])  [unwired: 1 in]
                n197 = Index Array(array=w464, index (row)=4) -> (element=w466:dbl[])  [unwired: 1 in]
                n198 = Index Array(array=w474, index=0) -> (element=w472:dbl)
                n199 = property class="DigNum (strict)"("Value"=w472) -> ()  [unwired: 2 in, 2 out]
                n200 = Index Array(array=w470, index=0) -> (element=w468:dbl)
                n201 = Index Array(array=w466, index=0) -> (element=w463:dbl)
                n202 = property on="Motor Control Loop Rate (ms)" class="DigNum (strict)"("Value"=w463) -> ()  [unwired: 2 in, 2 out]
                n203 = property on="Sensor Loop Rate (ms)" class="DigNum (strict)"("Value"=w468) -> ()  [unwired: 2 in, 2 out]
              }
            }
          }
          frame #1 {
          }
          frame #2 {
          }
        }
        n204 = Enqueue Element(queue=w460, element=enum16{"Start sensors", "load Values", "Idle"}."Idle" ("Enum")) -> (queue out=w459:refnum<queue>)  [unwired: 2 in, 2 out]
      }
      frame "Idle" {
        w481 = T2."Enabled" ("Disabled")
        n205 = event shown="[2] \"Start Sensors\": Value Change" {
          selector: _ -> [_ _ _]
          dyn-events: _ -> [_ _ _]
          timeout: _ -> [_ _ _]
          tunnel: w483 -> [w486 w489 w492]
          tunnel: [w485 w488 w491] -> w482
          event "Save Inputs": Value Change {
            n206 = event-data() -> ()  [unwired: 1 in, 6 out]
            n207 = Enqueue Element(queue=w486, element=enum16{"Start sensors", "load Values", "Idle"}."Idle" ("Enum")) -> (queue out=w485:refnum<queue>)  [unwired: 2 in, 2 out]
          }
          event "Load Inputs": Value Change {
            n208 = event-data() -> ()  [unwired: 1 in, 6 out]
            n209 = Enqueue Element(queue=w489, element=enum16{"Start sensors", "load Values", "Idle"}."Idle" ("Enum")) -> (queue out=w488:refnum<queue>)  [unwired: 2 in, 2 out]
          }
          event "Start Sensors": Value Change {
            n210 = event-data() -> ()  [unwired: 1 in, 6 out]
            n211 = Enqueue Element(queue=w492, element=enum16{"Start sensors", "load Values", "Idle"}."Start sensors" ("Enum")) -> (queue out=w491:refnum<queue>)  [unwired: 2 in, 2 out]
          }
        }
        n212 = property on="Start Sensors" class="Bool"("DisabledEnum"=w481) -> ()  [unwired: 2 in, 2 out]
        n213 = property on="Save Inputs" class="Bool"("DisabledEnum"=w481) -> ()  [unwired: 2 in, 2 out]
        n214 = property on="Load Inputs" class="Bool"("DisabledEnum"=w481) -> ()  [unwired: 2 in, 2 out]
        n215 = property on="Stop Sensors" class="Bool"("DisabledEnum"=T2."Disabled and Grayed Out" ("Disabled")) -> ()  [unwired: 2 in, 2 out]
      }
      frame "Start sensors" {
        w493 = 50.0
        w532 = T2."Disabled and Grayed Out" ("Disabled")
        # "threshold"
        # "Sensor Calibration and LabJack Read"
        n216 = Array Size(array=w524) -> (size(s)=w525:i32)
        n217 = property on="Stop Sensors" class="Bool"("DisabledEnum"=T2."Enabled" ("Disabled")) -> ()  [unwired: 2 in, 2 out]
        n218 = call "LJM_eReadNames.vi"("Handle In"=w530, "aNames"=string[] ["AIN0", "AIN3", "AIN2_EF_READ_A", "AIN4"], "error in"=w528) -> ("Handle Out"=w529:i32, "aValuesOut"=w520:dbl[], "error out"=w527:errorcluster)  [unwired: 9 in, 1 out]
        n219 = property on="Save Inputs" class="Bool"("DisabledEnum"=w532) -> ()  [unwired: 2 in, 2 out]
        n220 = property on="Start Sensors" class="Bool"("DisabledEnum"=w532) -> ()  [unwired: 2 in, 2 out]
        n221 = property on="Load Inputs" class="Bool"("DisabledEnum"=w532) -> ()  [unwired: 2 in, 2 out]
        n222 = for {
          N: w525 -> [_]
          tunnel: w524 -> [w554] mode=indexing
          tunnel: w523 -> [w555] mode=indexing
          tunnel: w520 -> [w557] mode=indexing
          tunnel: [w553] -> w509 mode=indexing
          n223 = Multiply(x=w555, y=w557) -> (x*y=w556:dbl)
          n224 = Add(x=w554, y=w556) -> (x+y=w553:dbl)
        }
        n225 = case shown="False" "Stop Sensors" {
          tunnel: w535 -> [w560 w563]
          tunnel: [w559 w562] -> w534
          frame False {
            n226 = Enqueue Element(queue=w560, element=enum16{"Start sensors", "load Values", "Idle"}."Start sensors" ("Enum")) -> (queue out=w559:refnum<queue>)  [unwired: 2 in, 2 out]
          }
          frame True {
            n227 = Enqueue Element(queue=w563, element=enum16{"Start sensors", "load Values", "Idle"}."Idle") -> (queue out=w562:refnum<queue>)  [unwired: 2 in, 2 out]
          }
        }
        n228 = Array Size(array=w509) -> (size(s)=w519:i32)
        n229 = Index Array(array=w509, index=T3."Potentiometer" ("labjacksInputs")) -> (element=w522:dbl)
        "Potentiometer distance" <- w522
        n230 = Index Array(array=w509, index=T3."Thermocouple" ("labjacksInputs")) -> (element=→"?" →"Stagnation Flow Temp (K)\n(For Refrence only)":dbl)
        n231 = for {
          N: w519 -> [_]
          tunnel: w509 -> [w552] mode=indexing
          tunnel: [w550] -> w518 mode=indexing
          n232 = Number To Decimal String(number=w552, width (-)=i16 5) -> (decimal integer string=w550:string)
        }
        n233 = Index Array(array=w509, index=T3."Ducer" ("labjacksInputs")) -> (element=w494:dbl)
        "Raw Pressure Ducer" <- w494
        n234 = Index Array(array=w509, index=T3."Ducer2" ("labjacksInputs")) -> (element=w496:dbl)
        "Raw Pressure Ducer 2" <- w496
        n235 = Subtract(x=w496, y=w494) -> (x-y=w507:dbl)
        n236 = Absolute Value(x=w507) -> (abs(x)=w506:dbl)
        n237 = Format Date/Time String(time format string (%c)="%H%M%S%3u") -> (date/time string=w513:string)  [unwired: 2 in]
        n238 = Insert Into Array(array=w518, new element=w513) -> (w517:string[])  [unwired: 1 in]
        n239 = Build Array (concatenate)(w517, w515) -> (w516:string[][])
        n240 = In Range and Coerce(upper limit=w493, x=w506, lower limit=w493) -> ()  [unwired: 2 out]
        n241 = Add(x=w496, y=w494) -> (x+y=w504:dbl)
        n242 = Divide(x=w504, y=2) -> (x/y=w495:dbl)
        n243 = event shown="[2] \"Use D1\": Value Change" {
          selector: _ -> [_ _ _]
          dyn-events: _ -> [_ _ _]
          timeout: _ -> [_ _ _]
          tunnel: [FALSE FALSE TRUE] -> w502
          tunnel: [FALSE TRUE FALSE] -> w501
          tunnel: [TRUE FALSE FALSE] -> w500
          event "Use Avg": Value Change {
            n244 = event-data() -> ()  [unwired: 1 in, 6 out]
          }
          event "Use D2": Value Change {
            n245 = event-data() -> ()  [unwired: 1 in, 6 out]
          }
          event "Use D1": Value Change {
            n246 = event-data() -> ()  [unwired: 1 in, 6 out]
          }
        }
        "Ducer2" <- w501
        "Ducer1" <- w502
        "Avg Ducers" <- w500
        n247 = case shown="False" "Use Avg" {
          tunnel: [w545 w549] -> w503
          tunnel: "Use D2" -> [_ _]
          tunnel: "Use D1" -> [w548 _]
          tunnel: w496 -> [w546 _]
          tunnel: w495 -> [_ w549]
          tunnel: w494 -> [w547 _]
          frame False {
            n248 = Select(t=w546, s=w548, f=w547) -> (s? t:f=w545:dbl)
          }
          frame True {
          }
        }
        "Read Pressure Ducer" <- w503
      }
    }
    n249 = Divide(x=w449, y=u32 1000) -> (x/y=→"Time Since Start (s)\n(For Reference Only)":dbl)
  }
  n250 = Release Queue(queue=w22) -> ()  [unwired: 2 in, 3 out]
  n251 = call "LJM_Close.vi"("error in"=w29, "Handle"=w28) -> ("error out"=→"Labjack error":errorcluster)  [unwired: 9 in]
  n252 = VISA Close(VISA resource name=w12, error in (no error)=w11) -> (error out=→"Arduino Error":errorcluster)
  n253 = Release Queue(queue=w21) -> ()  [unwired: 2 in, 3 out]
